vi "Init ECAT Reconfig VI.vi"(8 "error in (no error)":errorcluster, 11 "ECAT Modules":T2[](array[typedef])) -> (0 "error out":errorcluster, 3 "ECAT Reconfig out":T1)   [LabVIEW 2020, in "SEECD Engine.lvlib"]
uses:
  SEECD Engine.lvlib
  Type Defs/ECAT Reconfig State.ctl
  Type Defs/ECAT Reconfig Status.ctl
  Type Defs/ECAT Reconfig Data.ctl
  <vilib>/NI VeriStand/Custom Device Tools/Custom Device Utility Library/Custom Device Utility Library.lvlib
  Includes/Modules.lvlibp/RSI Module/RSI Module.lvclass
  Type Defs/ECAT Module Reconfig.ctl
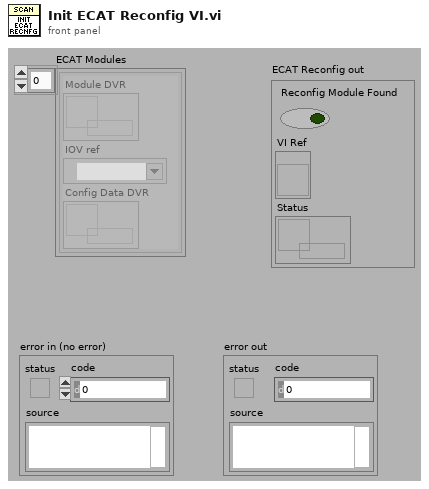
[diagram p1: front panel]
types:
  T1 = typedef "SEECD Engine.lvlib/ECAT Reconfig Data.ctl" = cluster{"Reconfig Module Found":bool, "VI Ref":refnum<vi>, "Status":refnum<queue>}
  T2 = typedef "SEECD Engine.lvlib/ECAT Module Reconfig.ctl" = cluster{"Module DVR":refnum<data-value>, "IOV ref":refnum<k21>, "Config Data DVR":refnum<data-value>}
  T3 = typedef "SEECD Engine.lvlib/ECAT Reconfig State.ctl" = enum16{"Not running", "Waiting to Start", "Started", "Running"}
  T4 = typedef "SEECD Engine.lvlib/ECAT Reconfig Status.ctl" = cluster{"State":T3, "error":errorcluster}
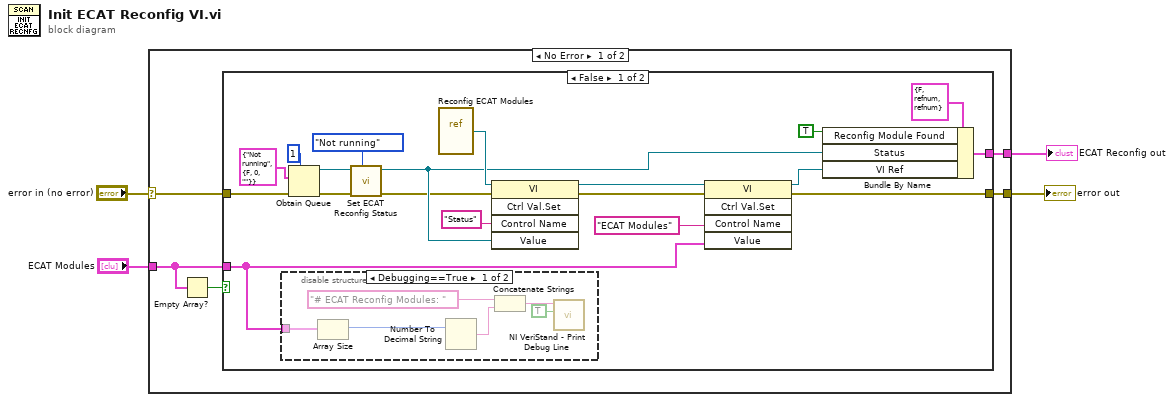
[diagram p0: block diagram]
diagram:
  n1 = case shown="No Error" "error in (no error)" {
    selector: "error in (no error)" -> [w9 w36]
    tunnel: "ECAT Modules" -> [w6 _]
    tunnel: [w8 w36] -> w4
    tunnel: [w5 _] -> w1
    frame No Error {
      n2 = Empty Array?(array=w6) -> (empty?=w7:bool)
      n3 = case shown="False" w7 {
        tunnel: w6 -> [w20 _]
        tunnel: w9 -> [w22 w35]
        tunnel: [w21 w35] -> w8
        tunnel: [w17 _] -> w5
        frame False {
          n4 = disable-structure shown="Debugging==True" {
            disable-tunnel: w20 -> [w32 _]
            frame condition #0 {
              n5 = Array Size(array=w32) -> (size(s)=w31:i32)
              n6 = Number To Decimal String(number=w31) -> (decimal integer string=w30:string)  [unwired: 1 in]
              n7 = Concatenate Strings("# ECAT Reconfig Modules: ", w30) -> (w33:string)
              n8 = call <vilib>:"NI VeriStand - Print Debug Line.vi"("Add to log file? (F)"=TRUE, "Message"=w33) -> ()  [unwired: 9 in, 1 out]
            }
            frame condition #1 (active) {
            }
          }
          n9 = Obtain Queue(max queue size (-1, unlimited)=1, element data type=T4 {"State"=enum."Not running", "error"={"status"=FALSE, "code"=0, "source"=""}} ("ECAT Reconfig Status"), error in (no error)=w22) -> (queue out=w10:refnum<queue>, error out=w15:errorcluster)  [unwired: 2 in, 1 out]
          n10 = call "Set ECAT Reconfig Status.vi"("State"=ECAT_Reconfig_State."Not running", "error in (no error)"=w15, "Status in"=w10) -> ("error out"=w12:errorcluster, "Status out"=w14:refnum<queue>)  [unwired: 7 in]
          n11 = vi-ref "Reconfig ECAT Modules.vi"() -> (w23:refnum<vi>)
          n12 = invoke class="VI" method="Ctrl Val.Set"(reference=w23, error in=w12, "Control Name"="Status", "Value"=w14) -> (reference out=w24:refnum<vi>, error out=w25:errorcluster)  [unwired: 1 in, 3 out]
          n13 = invoke class="VI" method="Ctrl Val.Set"(reference=w24, error in=w25, "Control Name"="ECAT Modules", "Value"=w20) -> (reference out=w16:refnum<vi>, error out=w21:errorcluster)  [unwired: 1 in, 3 out]
          n14 = Bundle By Name(cluster=T1 {"Reconfig Module Found"=FALSE, "VI Ref"=refnum, "Status"=refnum} ("ECAT Reconfig out"), "Reconfig Module Found"=TRUE, "Status"=w14, "VI Ref"=w16) -> (w17:T1)
        }
        frame True {
        }
      }
    }
    frame Error {
    }
  }
  "error out" <- w4
  "ECAT Reconfig out" <- w1
